vi "GEOM_SetupROIs.vi"(5 "FPAReadMode":T1 {"Amplifiers"."fliped" items=["none", "horizontal", "vertical"]; "Amplifiers"."type" items=["LL", "LR", "UL", "UR"]}, 7 "CorrectionType":T10, 8 "GEOM_modifiers":T6={"Binning"={"x"=1, "y"=1}, "sections"=[]} {"Binning"."y" min=1; "Binning"."x" min=1}, 9 "ROIs":T5[](array[typedef]), 10 "GEOM_FPAReadModes":T1[](array[typedef]) {"Amplifiers"."fliped" items=["none", "horizontal", "vertical"]; "Amplifiers"."type" items=["LL", "LR", "UL", "UR"]}) -> (1 "bin corr fpa":T9[](array[typedef]), 2 "nbincorr fpa":T9[](array[typedef]), 3 "GEOM_FPAReadModes  out":T1[](array[typedef]) {"Amplifiers"."fliped" items=["none", "horizontal", "vertical"]; "Amplifiers"."type" items=["LL", "LR", "UL", "UR"]})   [LabVIEW 2016]
uses:
  GEOM_ROICorrection.ctl
  GEOM_FPAReadMode.ctl
  GEOM_Amplifier.ctl
  GEOM_AmpType.ctl
  GEOM_ROI.ctl
  GEOM_Coords.ctl
  GEOM_CorrectedFPA.ctl
  GEOM_AmpModifiers.ctl
  GEOM_Binning.ctl
  GEOM_Moifier.ctl
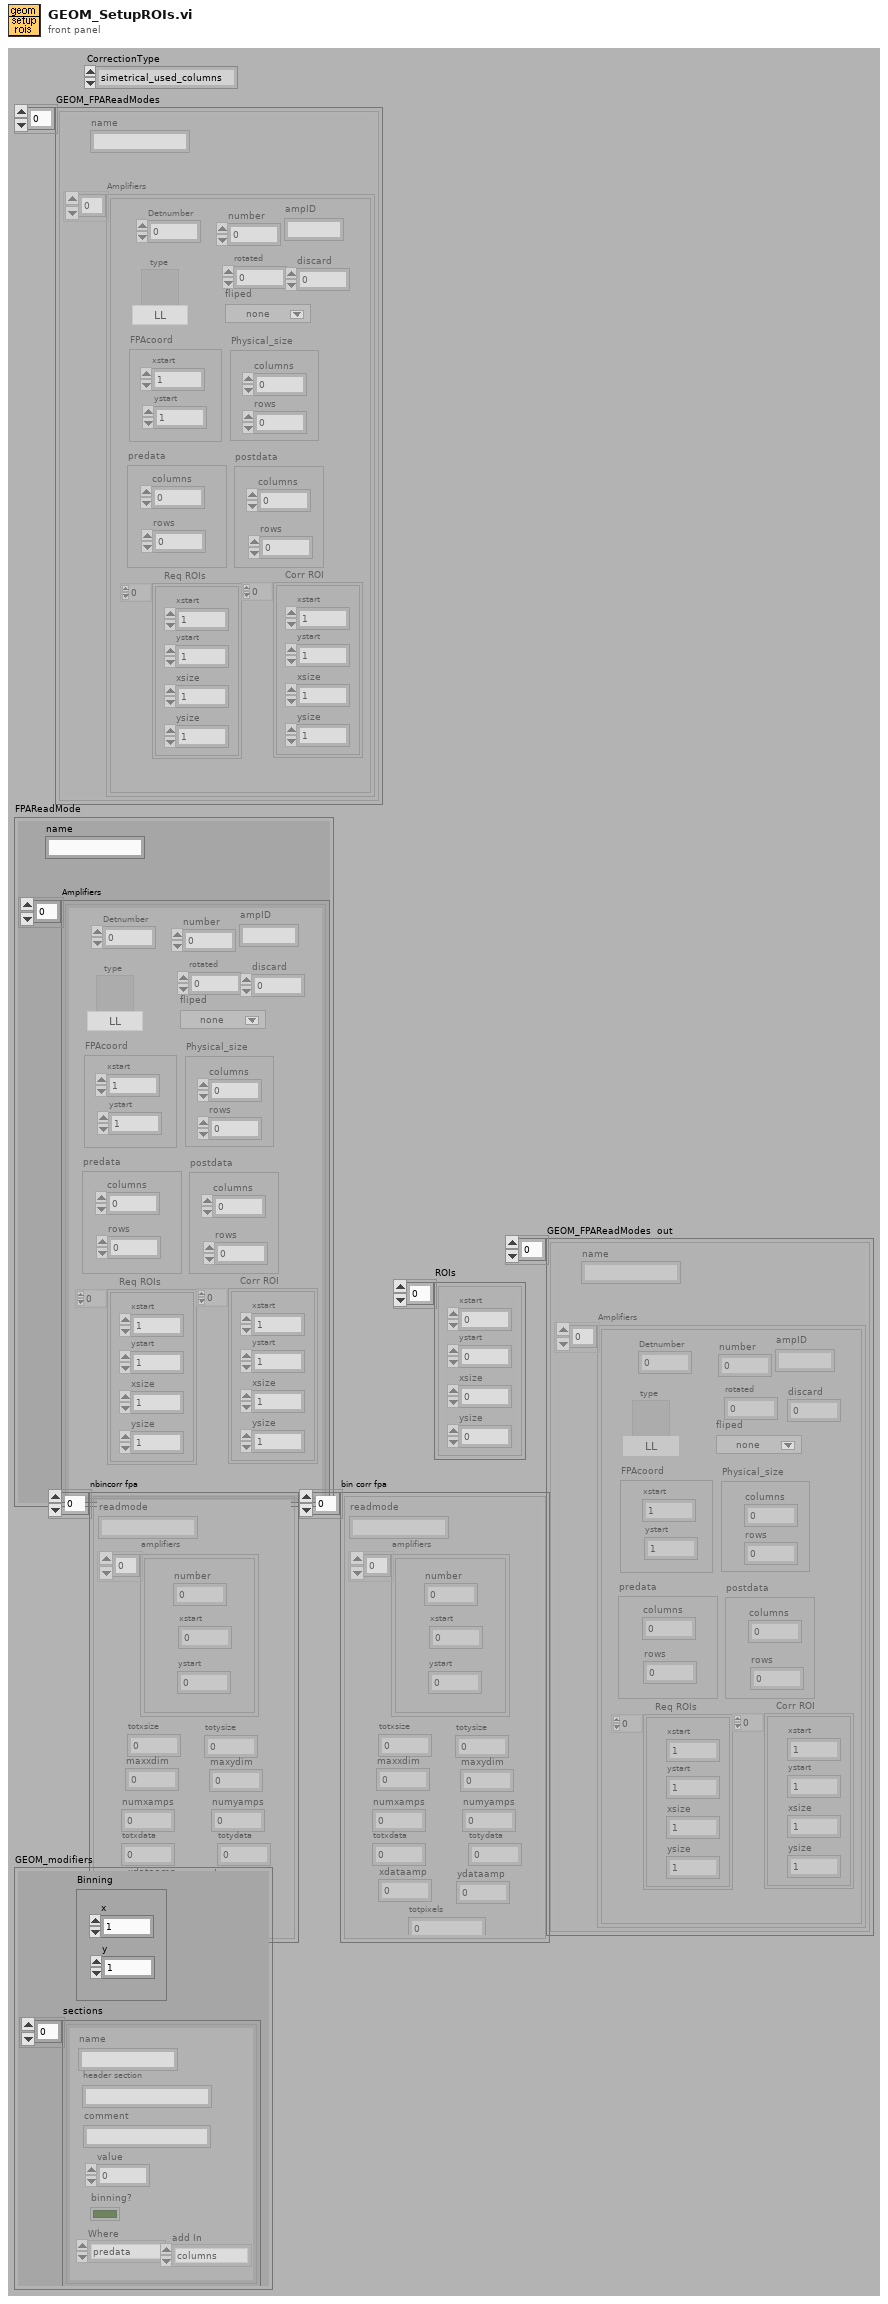
[diagram p1: front panel]
types:
  T1 = typedef "GEOM_FPAReadMode.ctl" = cluster{"name":string, "Amplifiers":T2[]}
  T2 = typedef "GEOM_Amplifier.ctl" = cluster{"number":i32, "type":T3, "rotated":i16, "fliped":u16, "FPAcoord":cluster{"xstart":i32, "ystart":i32}, "Physical_size":cluster{"columns":i32, "rows":i32}, "predata":cluster{"columns":i32, "rows":i32}, "postdata":cluster{"columns":i32, "rows":i32}, "Req ROIs":T4, "Corr ROI":T4, "Detnumber":i32, "ampID":string, "discard":i32}
  T3 = typedef "GEOM_AmpType.ctl" = u16
  T4 = typedef "GEOM_ROI.ctl" = T5[]
  T5 = typedef "GEOM_Coords.ctl" = cluster{"xstart":u32, "ystart":u32, "xsize":u32, "ysize":u32}
  T6 = typedef "GEOM_AmpModifiers.ctl" = cluster{"Binning":T7, "sections":T8[]}
  T7 = typedef "GEOM_Binning.ctl" = cluster{"x":u32, "y":u32}
  T8 = typedef "GEOM_Moifier.ctl" = cluster{"name":string, "header section":string, "comment":string, "value":i32, "binning?":bool, "Where":enum16{"predata", "postdata"}, "add In":enum16{"columns", "rows", "none"}}
  T9 = typedef "GEOM_CorrectedFPA.ctl" = cluster{"readmode":string, "amplifiers":cluster{"number":i32, "xstart":i32, "ystart":i32}[], "totxsize":i32, "totysize":i32, "maxxdim":i32, "maxydim":i32, "numxamps":i32, "numyamps":i32, "totxdata":i32, "totydata":i32, "xdataamp":i32, "ydataamp":i32, "totpixels":i32}
  T10 = typedef "GEOM_ROICorrection.ctl" = enum16{"simetrical_used_columns", "simetrical_all_columns"}
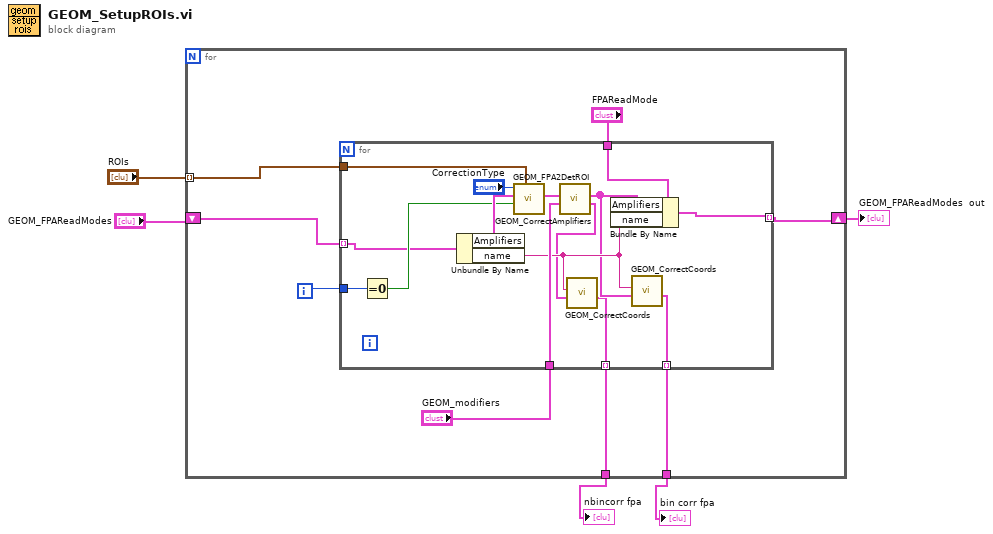
[diagram p0: block diagram]
diagram:
  n1 = for {
    shift-right: [w6] -> w1
    shift-left: "GEOM_FPAReadModes" -> [w7]
    tunnel: "ROIs" -> [w11] mode=indexing
    tunnel: [w10] -> w3
    tunnel: [w9] -> w2
    i -> [w8]
    n2 = for {
      tunnel: w11 -> [w28]
      tunnel: "FPAReadMode" -> [w26]
      tunnel: "GEOM_modifiers" -> [w24]
      tunnel: [w19] -> w9 mode=indexing
      tunnel: [w18] -> w10 mode=indexing
      tunnel: w8 -> [w17]
      tunnel: w7 -> [w14] mode=indexing
      tunnel: [w15] -> w6 mode=indexing
      n3 = Equal To 0?(x=w17) -> (x = 0?=w16:bool)
      n4 = Unbundle By Name(w14) -> ("Amplifiers"=w27:T2[], "name"=w22:string)
      n5 = call "GEOM_FPA2DetROI.vi"("ROIcoords"=w28, "clean first?"=w16, "amplifiers"=w27, "CorrectionType"="CorrectionType") -> ("amplifiers out"=w25:T2[])  [unwired: 7 out]
      n6 = call "GEOM_CorrectAmplifiers.vi"("modifiers"=w24, "Amplifiers"=w25) -> ("NonBinnedAmplifiers"=w20:T2[], "BinnedAmplifiers"=w21:T2[])  [unwired: 2 in, 6 out]
      n7 = call "GEOM_CorrectCoords.vi"("Amplifiers"=w20, "readmode"=w22) -> ("correctedReadMode"=w19:T9)  [unwired: 9 out]
      n8 = Bundle By Name(cluster=w26, "Amplifiers"=w21, "name"=w22) -> (w15:T1)
      n9 = call "GEOM_CorrectCoords.vi"("Amplifiers"=w21, "readmode"=w22) -> ("correctedReadMode"=w18:T9)  [unwired: 9 out]
    }
  }
  "bin corr fpa" <- w3
  "nbincorr fpa" <- w2
  "GEOM_FPAReadModes  out" <- w1
